vi "Get AI Data Value (By Name).vi"(6 "Raw? (false)":bool, 8 "error in (no error)":errorcluster, 9 "IOName (null)":variant, 10 "Name":string, 11 "DAQ":refnum<class "DAQ.lvclass">) -> (0 "error out":errorcluster, 1 "Timestamp (DBL)":dbl, 2 "Value":dbl, 3 "DAQ":refnum<class "DAQ.lvclass">, 5 "Time Stamp":timestamp)   [LabVIEW 2017, in "DAQ.lvclass"]
doc: "Developed by Kevin Thompson\nkevin@thompsonengineering.net\n\nCopyright 2018-2020\nThompson Engineering, LLC"
uses:
  DAQ.lvclass
  Process/ProcessSupport/TD DaqThread--enum.ctl
  DAQ.lvclass/DAQ.ctl
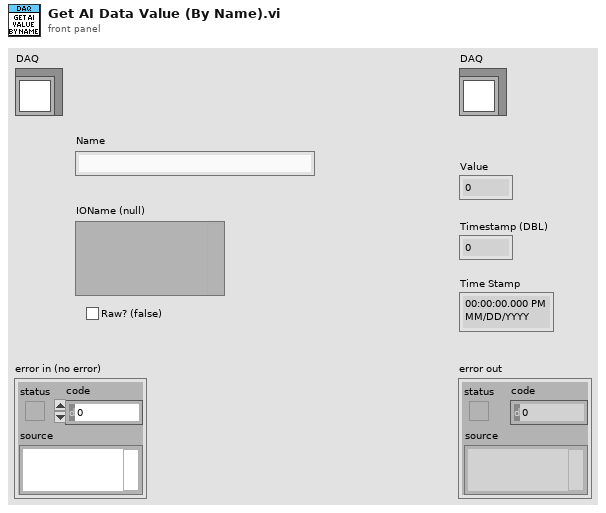
[diagram p1: front panel]
types:
  T1 = typedef "DAQ.lvclass/TD DaqThread--enum.ctl" = enum16{"AI", "DI"}
  T2 = typedef "TD Dynamic CVT DVR--ref.ctl" = refnum<data-value>
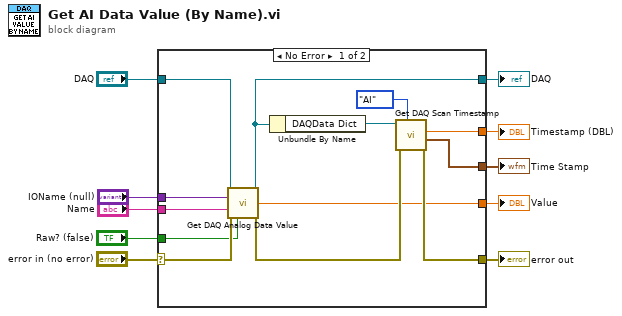
[diagram p0: block diagram]
diagram:
  n1 = case shown="No Error" "error in (no error)" {
    selector: "error in (no error)" -> [w23 w25]
    tunnel: [w18 w25] -> w9
    tunnel: [w21 w24] -> w7
    tunnel: "DAQ" -> [w22 w24]
    tunnel: [w16 _] -> w5
    tunnel: [w15 _] -> w6
    tunnel: [w14 _] -> w4
    tunnel: "Raw? (false)" -> [w13 _]
    tunnel: "IOName (null)" -> [w12 _]
    tunnel: "Name" -> [w11 _]
    frame No Error {
      n2 = call "Get DAQ Analog Data Value.vi"("DAQ"=w22, "IOName (enum)"=w12, "Name"=w11, "error in (no error)"=w23, "Raw? (false)"=w13) -> ("DAQ"=w21:refnum<class "DAQ.lvclass">, "Value"=w14:dbl, "error out"=w19:errorcluster)  [unwired: 8 in]
      n3 = Unbundle By Name(w21) -> ("DAQData Dict"=w20:T2)
      n4 = call "Get DAQ Scan Timestamp.vi"("Daq Thread"=TD_DaqThread--enum."AI", "error in (no error)"=w19, "DaqData dCVT"=w20) -> ("error out"=w18:errorcluster, "Time Stamp"=w15:timestamp, "Timestamp (DBL)"=w16:dbl)  [unwired: 5 in, 1 out]
    }
    frame Error {
    }
  }
  "error out" <- w9
  "DAQ" <- w7
  "Value" <- w4
  "Time Stamp" <- w6
  "Timestamp (DBL)" <- w5
